vi "Transceiver Thread.Get Transfer Group.vi"(10 "index":i32, 11 "Transceiver Thread in":refnum<class "Transceiver Thread.lvclass">) -> (2 "Transfer Group":refnum<class "Transfer Group.lvclass">, 3 "Transceiver Thread out":refnum<class "Transceiver Thread.lvclass">)   [LabVIEW 2017, in "DSF.Engine.lvlib" / "Transceiver Thread.lvclass"]
uses:
  Transceiver Thread.lvclass
  Transfer/Transfer Group.lvclass
  Transceiver Thread.lvclass/Transceiver Thread.ctl
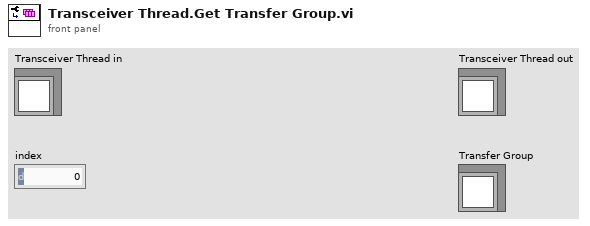
[diagram p1: front panel]
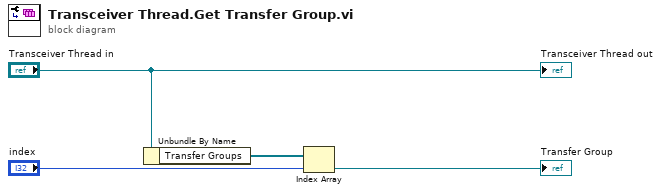
[diagram p0: block diagram]
diagram:
  n1 = Unbundle By Name("Transceiver Thread in") -> ("Transfer Groups"=w3:refnum<class "Transfer Group.lvclass">[])
  n2 = Index Array(array=w3, index="index") -> (element=→"Transfer Group":refnum<class "Transfer Group.lvclass">)
  "Transceiver Thread out" <- "Transceiver Thread in"
